vi "WPI_CANJaguar_AddConfigMessage.vi"(9 "Data":u8[](array[numeric]) format="%.0x", 10 "Message ID":u32, 11 "CAN Jaguar Ref":T1={"DeviceStatus"={"status"=FALSE, "code"=0, "source"=""}, "Type"=enum."PWM", "PWM"={"PWM Channel"=enum."PWM 1", "DeadBand"={"Name"="", "maxPositivePwm"=0, "minPositivePwm"=0, "centerPwm"=0, "maxNegativePwm"=0, "minNegativePwm"=0, "angularRange"=0}}, "CAN"={"Device Number"=0, "SetOutput VI Ref"=variant(enum8{"Percent VBus", "Current", "Speed", "Position", "Voltage"} enum."Percent VBus"), "GetOutput VI Ref"=variant(refnum<k1> refnum), "Enable VI Ref"=variant(dbl 12.0), "Disable VI Ref"=variant(enum8{"Percent VBus", "Speed", "Position", "Slave", "Unchanged / Invalid", "Voltage Compensation", "Current", "Motion Profile"} enum."Percent VBus"), "Data"=variant}, "Invert"=FALSE}) -> ()   [LabVIEW 2016]
uses:
  <vilib>/Rock Robotics/WPI/MotorControl/WPI_MotorControlDeviceRef.ctl
  <vilib>/Rock Robotics/WPI/MotorControl/WPI_MotorControlType.ctl
  <vilib>/Rock Robotics/SystemInterfaces/DIO/FPGA_DIOPWMChannel.ctl
  <vilib>/Rock Robotics/WPI/PWM/WPI_PWMDeadband.ctl
  <vilib>/Rock Robotics/WPI/ThirdParty/CanMotor/CAN Jaguar/SubVIs/WPI_CANJaguar_ConfigMessage.ctl
  <vilib>/Rock Robotics/WPI/ThirdParty/CanMotor/CAN Jaguar/SubVIs/WPI_CAN_TokenMessageIDs.ctl
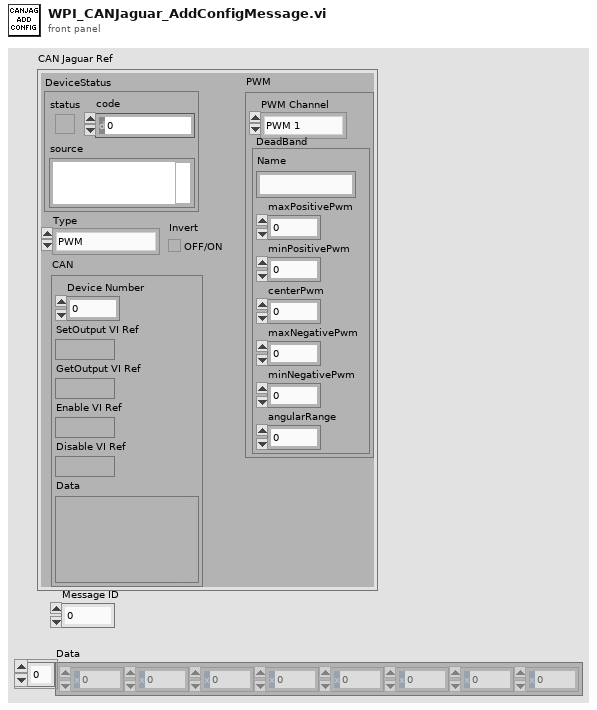
[diagram p1: front panel]
types:
  T1 = typedef "WPI_MotorControlDeviceRef.ctl" = cluster{"DeviceStatus":errorcluster, "Type":T2, "PWM":cluster{"PWM Channel":T3, "DeadBand":T4}, "CAN":cluster{"Device Number":u8, "SetOutput VI Ref":variant, "GetOutput VI Ref":variant, "Enable VI Ref":variant, "Disable VI Ref":variant, "Data":variant}, "Invert":bool}
  T2 = typedef "WPI_MotorControlType.ctl" = enum16{"PWM", "CAN"}
  T3 = typedef "FPGA_DIOPWMChannel.ctl" = enum8{"PWM 0", "PWM 1", "PWM 2", "PWM 3", "PWM 4", "PWM 5", "PWM 6", "PWM 7", "PWM 8", "PWM 9", "PWM MXP 0", "PWM MXP 1", "PWM MXP 2", "PWM MXP 3", "PWM MXP 4", "PWM MXP 5", "PWM MXP 6", "PWM MXP 7", "PWM MXP 8", "PWM MXP 9", "Invalid"}
  T4 = typedef "WPI_PWMDeadband.ctl" = cluster{"Name":string, "maxPositivePwm":i32, "minPositivePwm":i32, "centerPwm":i32, "maxNegativePwm":i32, "minNegativePwm":i32, "angularRange":u16}
  T5 = typedef "WPI_CAN_TokenMessageIDs.ctl" = u32
  T6 = typedef "WPI_CANJaguar_ConfigMessage.ctl" = cluster{"Message ID":u32, "Needs Check":bool, "Data":u8[], "Mode":bool}
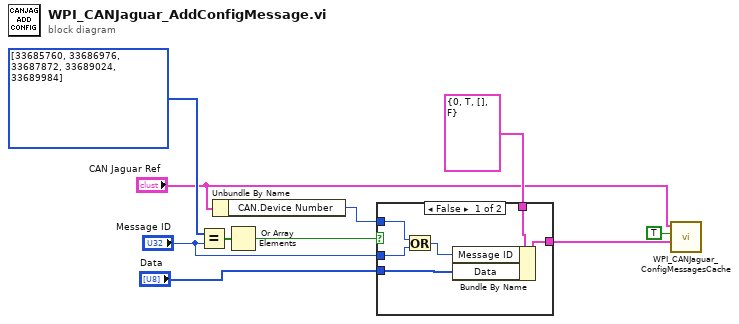
[diagram p0: block diagram]
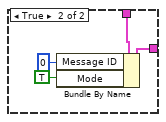
[diagram p2: hidden frame]
diagram:
  w6 = T5[] [33685760, 33686976, 33687872, 33689024, 33689984] items=["Token Volt Enable"=33685760, "Token Volt Set"=33685824, "Token Volt Set No Ack"=33685952, "Token Speed Enable"=33686976, "Token Speed Set"=33687040, "Token Speed Set No Ack"=33687168, "Token Volt Comp Enable"=33687872, "Token Volt Comp Set"=33687936, "Token Volt Comp Set No Ack"=33688064, "Token Position Enable"=33689024, "Token Position Set"=33689088, "Token Position Set No Ack"=33689216, "Token Current Enable"=33689984, "Token Current Set"=33690048, "Token Current Set No Ack"=33690176]
  n1 = Equal?(x=w6, y="Message ID") -> (x = y?=w4:bool[])
  n2 = Unbundle By Name("CAN Jaguar Ref") -> ("CAN.Device Number"=w1:u8)
  n3 = Or Array Elements(Boolean array=w4) -> (logical OR=w3:bool)
  n4 = case shown="False" w3 {
    tunnel: T6 {"Message ID"=0, "Needs Check"=TRUE, "Data"=[], "Mode"=FALSE} ("Config Message") -> [w16 w20]
    tunnel: [w15 w19] -> w8
    tunnel: "Data" -> [w14 _]
    tunnel: "Message ID" -> [w12 _]
    tunnel: w1 -> [w13 _]
    frame False {
      n5 = Or(x=w13, y=w12) -> (x .or. y?=w11:u32)
      n6 = Bundle By Name(cluster=w16, "Message ID"=w11, "Data"=w14) -> (w15:T6)
    }
    frame True {
      n7 = Bundle By Name(cluster=w20, "Message ID"=u32 0, "Mode"=TRUE) -> (w19:T6)
    }
  }
  n8 = call <vilib>:"WPI_CANJaguar_ConfigMessagesCache.vi"("Config Message"=w8, "Update"=TRUE, "CAN Jaguar Ref"="CAN Jaguar Ref") -> ()  [unwired: 8 in, 1 out]
